vi "Fare-Cel.vi"() -> ()   [LabVIEW 2024]
panel:
  out "Numeric 2":dbl
  in  "Numeric":dbl
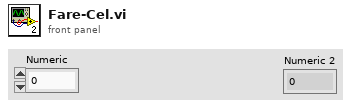
[diagram p1: front panel]
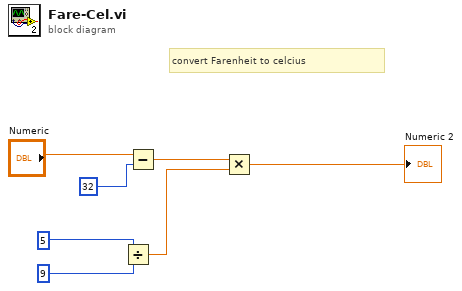
[diagram p0: block diagram]
diagram:
  # "convert Farenheit to celcius"
  n1 = Divide(x=5, y=9) -> (x/y=w7:dbl)
  n2 = Subtract(x="Numeric", y=32) -> (x-y=w1:dbl)
  n3 = Multiply(x=w1, y=w7) -> (x*y=→"Numeric 2":dbl)
